vi "Test Vererbung.vi"() -> ()   [LabVIEW 2020]
uses:
  Adresse.ctl
  Steuerung PNS.lvclass
  SteuerungsType (Enum).ctl
  mini8 Steuerung PNS/mini8 Steuerung PNS.lvclass
  Schneider Steuerung PNS/Schneider Steuerung PNS.lvclass
panel:
  out "Istwerte 3":u16[](array[numeric])
  out "Istwerte 2":u16[](array[numeric])
  out "Istwerte":u16[](array[numeric])
  out "error out":errorcluster caption="Fehler (Ausgang)"
  out "SteuerungsType":T1
  out "Steuerung PNS (Ausgang)":refnum<class "Steuerung PNS.lvclass">
  out "Adressen out 2":T2
  out "Adressen out":T2
  out "Adressen":cluster{i32[][], i32}
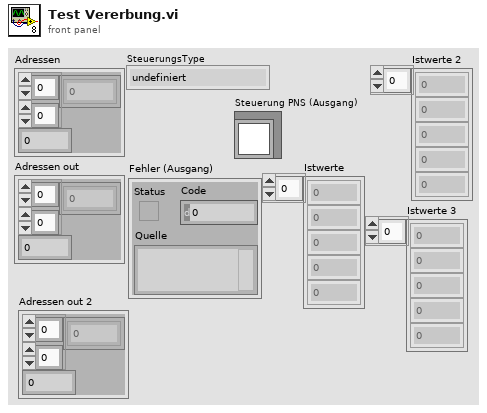
[diagram p1: front panel]
types:
  T1 = typedef "Steuerung PNS.lvclass/SteuerungsType (Enum).ctl" = enum16{"undefiniert", "Mini 8", "Schneider"}
  T2 = typedef "Steuerung PNS.lvclass/Adresse.ctl" = cluster{i32[][], i32}
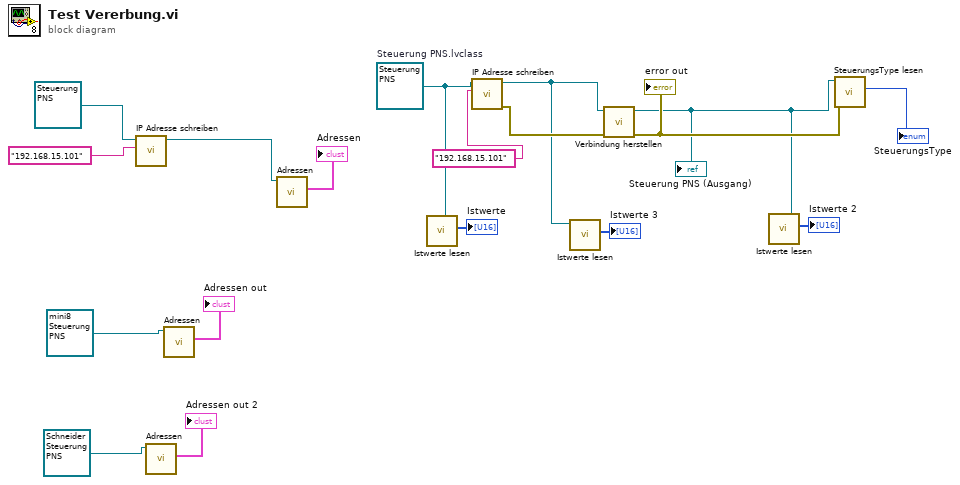
[diagram p0: block diagram]
diagram:
  w6 = refnum<class "Steuerung PNS.lvclass"> refnum  # Steuerung PNS.lvclass
  n1 = call-dynamic "IP Adresse schreiben.vi"("IP Adresse"="192.168.15.101" ("IP-Adresse"), "Steuerung PNS (Eingang)"=refnum<class "Steuerung PNS.lvclass"> refnum ("Steuerung PNS.lvclass")) -> ("Steuerung PNS (Ausgang)"=w16:refnum<class "Steuerung PNS.lvclass">)  [unwired: 8 in, 1 out]
  n2 = call-dynamic "Adressen.vi"("Schneider Steuerung PNS Eingang"=refnum<class "Schneider Steuerung PNS.lvclass"> refnum ("Schneider Steuerung PNS.lvclass")) -> ("Adressen out"=→"Adressen out 2":T2)  [unwired: 8 in, 2 out]
  n3 = call-dynamic "Adressen.vi"("mini8 Steuerung PNS Eingang"=refnum<class "mini8 Steuerung PNS.lvclass"> refnum ("mini8 Steuerung PNS.lvclass")) -> ("Adressen out"=→"Adressen out":T2)  [unwired: 8 in, 2 out]
  n4 = call-dynamic "Adressen.vi"("Steuerung PNS (Eingang)"=w16) -> ("Adressen"=→"Adressen":cluster{i32[][], i32})  [unwired: 8 in, 2 out]
  n5 = call-dynamic "Istwerte lesen.vi"("Steuerung PNS (Eingang)"=w6) -> ("Istwerte"=→"Istwerte":u16[])  [unwired: 8 in, 2 out]
  n6 = call-dynamic "IP Adresse schreiben.vi"("IP Adresse"="192.168.15.101" ("IP-Adresse"), "Steuerung PNS (Eingang)"=w6) -> ("error out"=w7:errorcluster, "Steuerung PNS (Ausgang)"=w2:refnum<class "Steuerung PNS.lvclass">)  [unwired: 8 in]
  n7 = call-dynamic "Istwerte lesen.vi"("Steuerung PNS (Eingang)"=w2) -> ("Istwerte"=→"Istwerte 3":u16[])  [unwired: 8 in, 2 out]
  n8 = call "Verbindung herstellen.vi"("error in (no error)"=w7, "Steuerung PNS (Eingang)"=w2) -> ("error out"=w9:errorcluster, "Steuerung PNS (Ausgang)"=w4:refnum<class "Steuerung PNS.lvclass">)  [unwired: 8 in]
  "Steuerung PNS (Ausgang)" <- w4
  "error out" <- w9
  n9 = call-dynamic "Istwerte lesen.vi"("Steuerung PNS (Eingang)"=w4) -> ("Istwerte"=→"Istwerte 2":u16[])  [unwired: 8 in, 2 out]
  n10 = call-dynamic "SteuerungsType lesen.vi"("error in (no error)"=w9, "Steuerung PNS (Eingang)"=w4) -> ("SteuerungsType"=→"SteuerungsType":T1)  [unwired: 7 in, 2 out]
